vi "点到行列.vi"(8 "错误输入（无错误）":errorcluster, 10 "点":T1 caption="表格点", 11 "引用":refnum<vi>) -> (0 "错误输出":errorcluster, 2 "单元格位置":T2 caption="表格位置", 3 "引用输出":refnum<vi>)   [LabVIEW 2014, in "表格.lvlib"]
uses:
  <vilib>/Utility/miscctls.llb/LVRowAndColumnTypeDef.ctl
  <vilib>/Utility/miscctls.llb/LVPositionTypeDef.ctl
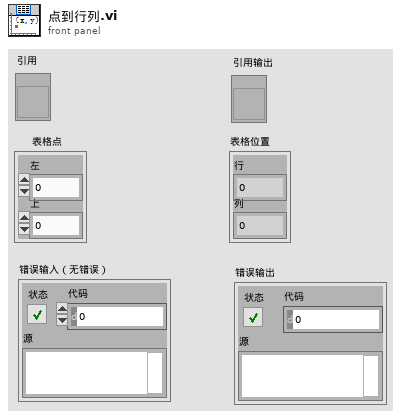
[diagram p1: front panel]
types:
  T1 = typedef "LVPositionTypeDef.ctl" = cluster{"Left":i32, "Top":i32}
  T2 = typedef "LVRowAndColumnTypeDef.ctl" = cluster{"Row":i32, "Column":i32}
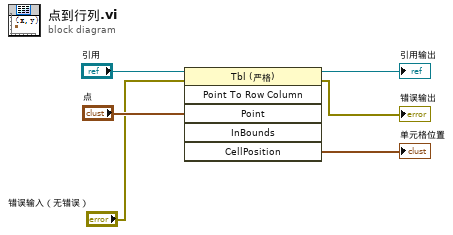
[diagram p0: block diagram]
diagram:
  n1 = invoke on="调用节点" class="Tbl (严格)" method="Point To Row Column"(reference="引用", error in="错误输入（无错误）", "Point"="点") -> (reference out=→"引用输出":refnum<vi>, error out=→"错误输出":errorcluster, "CellPosition"=→"单元格位置":T2)  [unwired: 3 in, 3 out]
